vi "Configure Number of Points.vi"(8 "error in (no error)":errorcluster, 10 "Number of Point":i32, 11 "VNA-Keysight PNA in":refnum<class "VNA-Keysight PNA.lvclass">) -> (0 "error out":errorcluster, 3 "VNA-Keysight PNA out":refnum<class "VNA-Keysight PNA.lvclass">)   [LabVIEW 2020, in "VNA-Keysight PNA.lvclass"]
doc: "Configures the number of points in the sweep.\nThe number of points will be choosen to the nearest supported."
uses:
  VNA-Keysight PNA.lvclass
  C:/Sandbox/Git_Sandbox/WiSpry Test Framework source code (LV20)/WiSpry Test Framework/Instruments/Instrument.lvclass
  Instrument.lvclass/Instrument.ctl
  Instrument.lvclass
  <instrlib>/Keysight PNA Series/Keysight PNA Series.lvlib
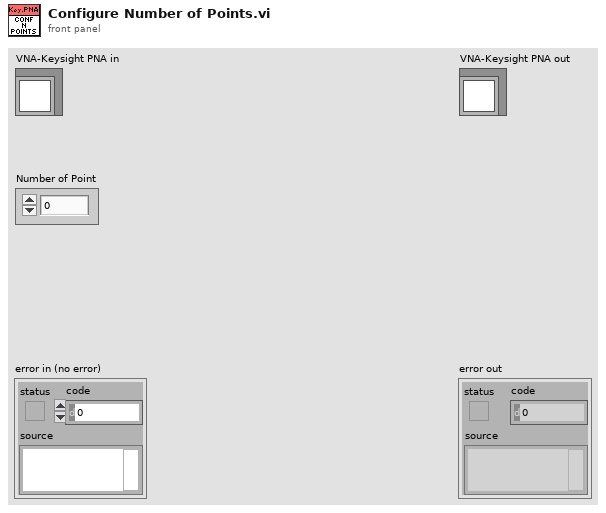
[diagram p1: front panel]
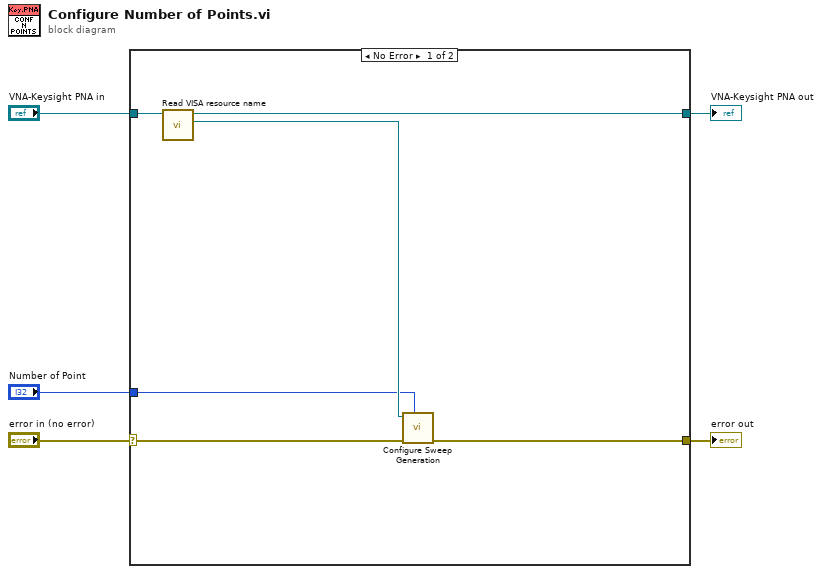
[diagram p0: block diagram]
diagram:
  n1 = case shown="No Error" "error in (no error)" {
    selector: "error in (no error)" -> [w9 w12]
    tunnel: [w10 w13] -> w4
    tunnel: "VNA-Keysight PNA in" -> [w11 w13]
    tunnel: [w8 w12] -> w5
    tunnel: "Number of Point" -> [w6 _]
    frame No Error {
      n2 = call "Read VISA resource name.vi"("Instrument in"=w11) -> ("VISA resource name"=w7:refnum<visa-resource-name>, "Instrument out"=w10:refnum<class "VNA-Keysight PNA.lvclass">)  [unwired: 9 in]
      n3 = call <instrlib>:"Configure Sweep Generation.vi"("Sweep Points (201)"=w6, "error in (no error)"=w9, "VISA resource name"=w7) -> ("error out"=w8:errorcluster)  [unwired: 7 in, 1 out]
    }
    frame Error {
    }
  }
  "error out" <- w5
  "VNA-Keysight PNA out" <- w4
